vi "CLD 7 Time Stamp to Initialization String exercise.vi"(8 "Error In":errorcluster) -> (0 "Error Out":errorcluster, 3 "Code String Out":string)   [LabVIEW 2025]
doc: "CLD 7 exercise"
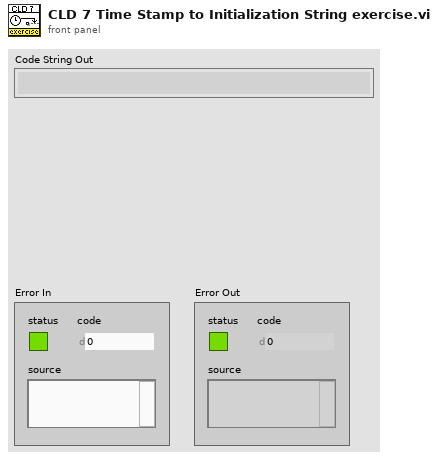
[diagram p1: front panel]
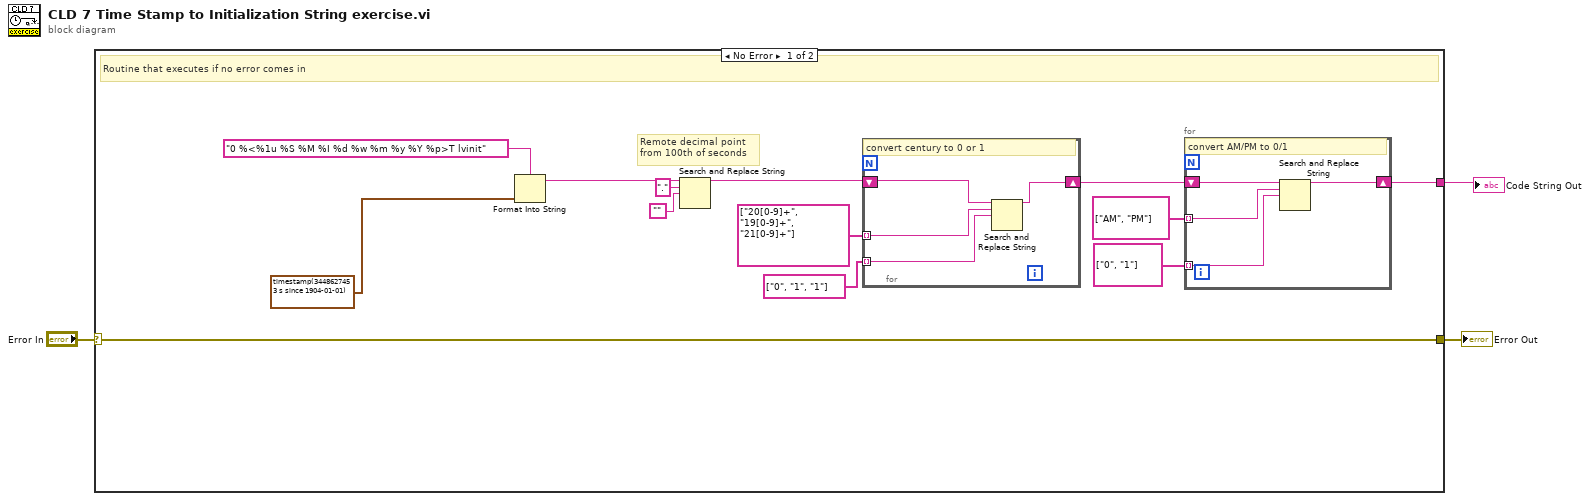
[diagram p0: block diagram]
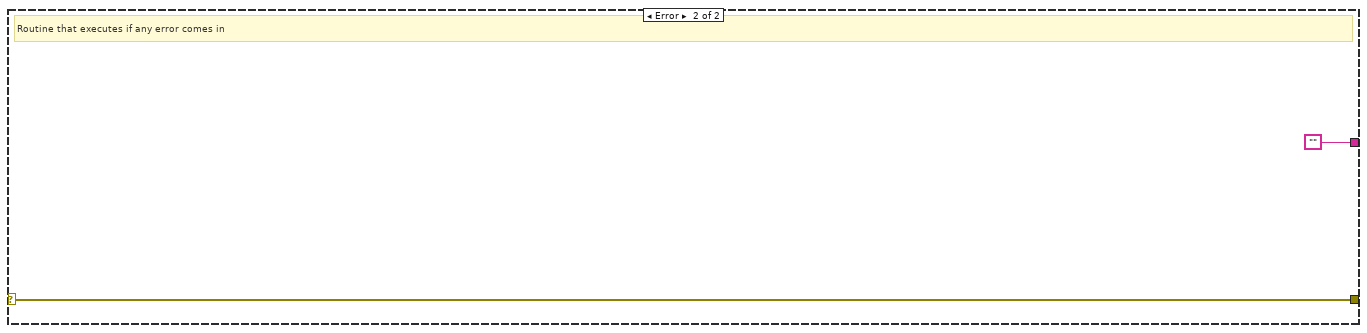
[diagram p2: hidden frame]
diagram:
  n1 = case shown="No Error" "Error In" {
    selector: "Error In" -> [w16 w26]
    tunnel: [w16 w26] -> w2
    tunnel: [w7 ""] -> w1
    frame No Error {
      # "Remote decimal point\nfrom 100th of seconds"
      # "Routine that executes if no error comes in"
      n2 = Format Into String(format string="0 %<%1u %S %M %I %d %w %m %y %Y %p>T lvinit", timestamp(3448627453 s since 1904-01-01) ("input 6")) -> (resulting string=w14:string)  [unwired: 2 in, 1 out]
      n3 = Search and Replace String(input string=w14, search string=".", replace string="") -> (result string=w13:string)  [unwired: 5 in, 3 out]
      n4 = for {
        shift-right: [w23] -> w8
        shift-left: w13 -> [w24]
        tunnel: string[] ["20[0-9]+", "19[0-9]+", "21[0-9]+"] ("input string") -> [w22] mode=indexing
        tunnel: string[] ["0", "1", "1"] ("replace string (\"\")") -> [w21] mode=indexing
        # "convert century to 0 or 1"
        n5 = Search and Replace String(input string=w24, search string=w22, replace string=w21) -> (result string=w23:string)  [unwired: 5 in, 3 out]
      }
      n6 = for {
        shift-right: [w19] -> w7
        shift-left: w8 -> [w20]
        tunnel: string[] ["AM", "PM"] -> [w18] mode=indexing
        tunnel: string[] ["0", "1"] -> [w17] mode=indexing
        # "convert AM/PM to 0/1"
        n7 = Search and Replace String(input string=w20, search string=w18, replace string=w17) -> (result string=w19:string)  [unwired: 5 in, 3 out]
      }
    }
    frame Error {
      # "Routine that executes if any error comes in"
    }
  }
  "Code String Out" <- w1
  "Error Out" <- w2
